vi "AddWorksheetFromExcelFile.vi"(8 "error in (no error)":errorcluster, 9 "Worksheet Name":string, 10 "ExcelFile To Copy From":refnum<class "PortableExcelFileManipulationOXML.lvclass">, 11 "ExcelFile in":refnum<class "PortableExcelFileManipulationOXML.lvclass">) -> (0 "error out":errorcluster, 3 "ExcelFile out":refnum<class "PortableExcelFileManipulationOXML.lvclass">)   [LabVIEW 2019, in "PortableExcelFileManipulationOXML.lvclass"]
doc: "Adds a worksheet to the This excel File by name."
uses:
  PortableExcelFileManipulationOXML.lvclass
  PortableExcelFileManipulationOXML.lvclass/PortableExcelFileManipulationOXML.ctl
  H:/LV projects/ExpressionEvaluator/Excel/ExcelManipulation.dll
  ExcelManipulation.dll
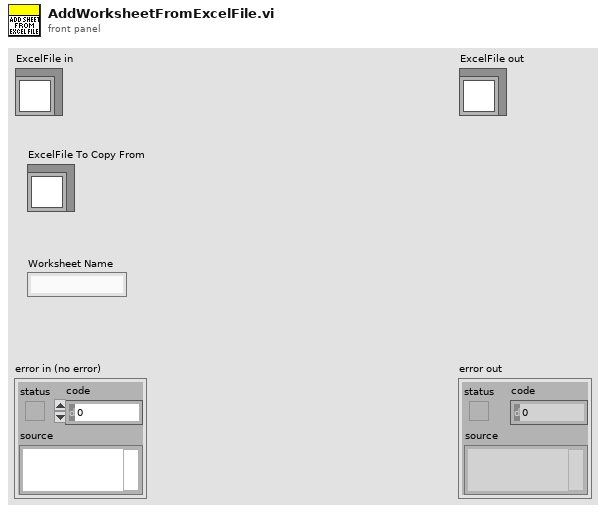
[diagram p1: front panel]
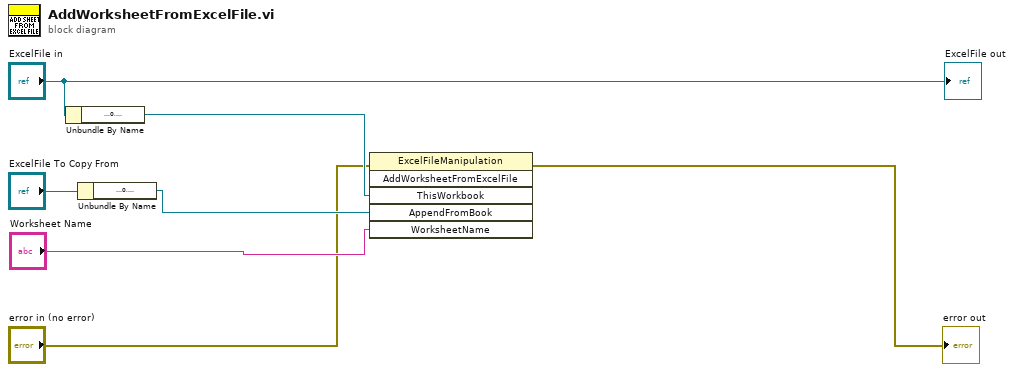
[diagram p0: block diagram]
diagram:
  n1 = Unbundle By Name("ExcelFile in") -> ("ExcelOpen"=w5:refnum<k24>)
  n2 = Unbundle By Name("ExcelFile To Copy From") -> ("ExcelOpen"=w4:refnum<k24>)
  n3 = invoke class="ExcelFileManipulation" method="AddWorksheetFromExcelFile"(error in="error in (no error)", "ThisWorkbook"=w5, "AppendFromBook"=w4, "WorksheetName"="Worksheet Name") -> (error out=→"error out":errorcluster)  [unwired: 2 in, 5 out]
  "ExcelFile out" <- "ExcelFile in"
